vi "PH_Sequencer.contents.vi"   [LabVIEW 2014, in "PH_Sequencer.lvlib"]
doc: "The Sequencer controlles the PHELIX shot procedure.\n\nThis class is part of the PHELIX user layer."
uses:
  PH_Sequencer.lvlib
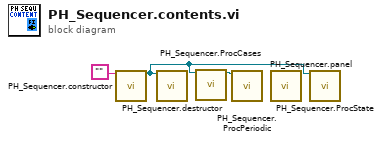
[diagram p0: block diagram]
diagram:
  n1 = call "PH_Sequencer.constructor.vi"("name"="") -> ("i ref out"=w1:refnum<vi>)  [unwired: 16 in, 2 out]
  n2 = call "PH_Sequencer.destructor.vi"("i ref in"=w1) -> ()  [unwired: 18 in, 1 out]
  n3 = call "PH_Sequencer.ProcCases.vi"("i ref in"=w1) -> ("i ref out"=w3:refnum<vi>)  [unwired: 16 in, 2 out]
  n4 = call "PH_Sequencer.ProcPeriodic.vi"("i ref in"=w3) -> ()  [unwired: 16 in, 3 out]
  n5 = call "PH_Sequencer.panel.vi"() -> ()  [unwired: 1 in]
  n6 = call "PH_Sequencer.ProcState.vi"("i ref in"=w1) -> ()  [unwired: 16 in, 3 out]
